vi "pc_pick2.vi"(0 "original array":i32[](array[numeric])) -> (1 "reduced array":i32[](array[numeric]), 2 "stack element 0":i32, 3 "stack element 1":i32)   [LabVIEW 2009]
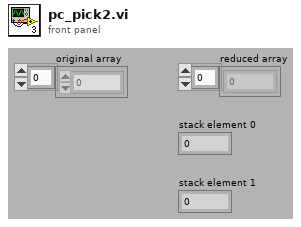
[diagram p1: front panel]
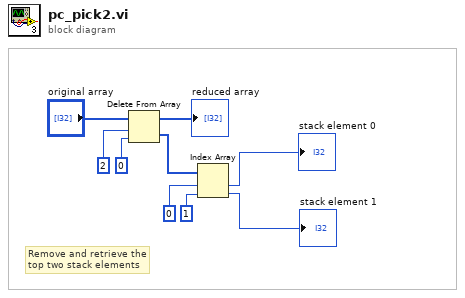
[diagram p0: block diagram]
diagram:
  # "Remove and retrieve the\ntop two stack elements"
  n1 = Delete From Array(array="original array", length=2 ("Länge"), index=0 ("Index")) -> (deleted portion=w5:i32[], array with subset deleted=→"reduced array":i32[])
  n2 = Index Array(array=w5, index #1=0 ("Index"), index #2=1 ("Index")) -> (element #1=→"stack element 0":i32, element #2=→"stack element 1":i32)
